vi "Func_StoreIconInfo.vi"() -> (2 "Text":T1[](array[typedef]) {"Body Text Spec"."Alignment" items=["left", "center", "right"]}, 3 "Layers":cluster{"User Layers":T5[]}[](array[cluster]) {"User Layers"."Data"."Opacity" scale=0.0..100.0})   [LabVIEW 2013]
uses:
  <vilib>/Utility/miscctls.llb/LVPoint32TypeDef.ctl
  IconEditorBuilds/2011IconEditor.llb/LayerType.ctl
  IconEditorBuilds/2011IconEditor.llb/Layer.ctl
  IconEditorBuilds/2011IconEditor.llb/User layer data.ctl
  TemplateGenerator.lvlib
  IconEditorBuilds/2011IconEditor.llb/GET Icon Text layer (VI).vi
  IconEditorBuilds/2011IconEditor.llb/GET Icon user layer (VI).vi
  IconEditorBuilds/2011IconEditor.llb/BodyText.ctl
  IconEditorBuilds/2011IconEditor.llb/Font Size.ctl
  IconEditorBuilds/2011IconEditor.llb/Alignment.ctl
  IconEditorBuilds/2011IconEditor.llb/Font.ctl
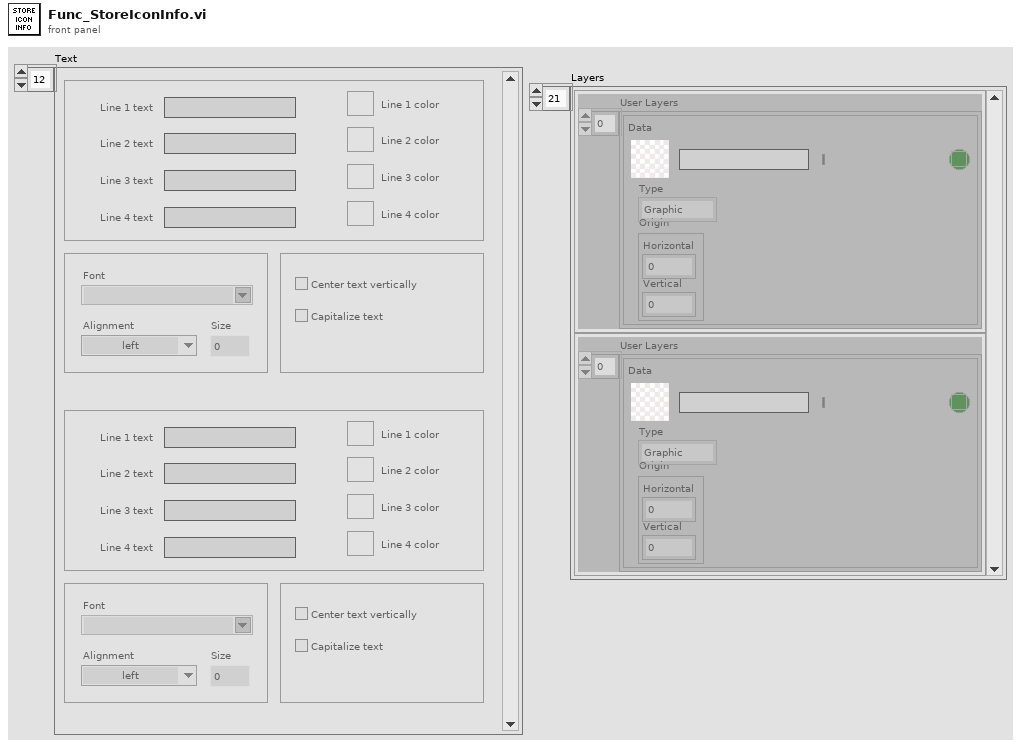
[diagram p1: front panel]
types:
  T1 = typedef "TemplateGenerator.lvlib/BodyText.ctl" = cluster{"Line 1 text":string, "Line 2 text":string, "Line 3 text":string, "Line 4 text":string, "Line 1 color":u32, "Line 2 color":u32, "Line 3 color":u32, "Line 4 color":u32, "Body Text Spec":cluster{"Font":T2, "Alignment":T3, "Size":T4}, "Center text vertically":bool, "Capitalize Text":bool}
  T2 = typedef "TemplateGenerator.lvlib/Font.ctl" = string
  T3 = typedef "TemplateGenerator.lvlib/Alignment.ctl" = u16
  T4 = typedef "TemplateGenerator.lvlib/Font Size.ctl" = u8
  T5 = typedef "TemplateGenerator.lvlib/2011 Icon Editor API.lvlib/User layer data.ctl" = cluster{"Data":T6, "Type":T7, "Origin":T8}
  T6 = typedef "TemplateGenerator.lvlib/Layer.ctl" = cluster{"LayerIcon":picture, "LayerName":string, "Opacity":u8, "Visibility?":bool}
  T7 = typedef "TemplateGenerator.lvlib/LayerType.ctl" = enum16{"Graphic", "Text", "Tool", "Graphic Drop"}
  T8 = typedef "LVPoint32TypeDef.ctl" = cluster{"Horizontal":i32, "Vertical":i32}
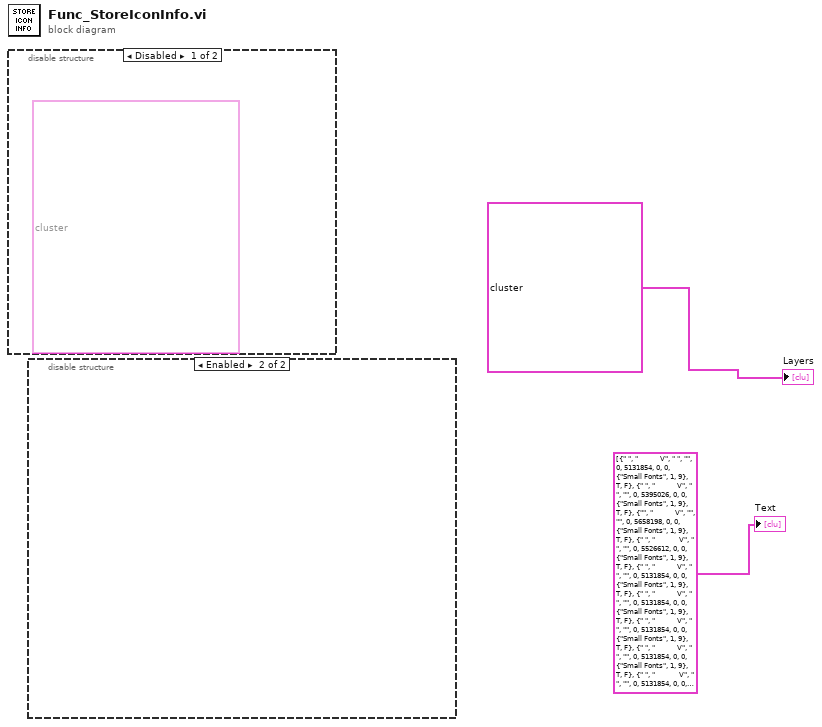
[diagram p0: block diagram]
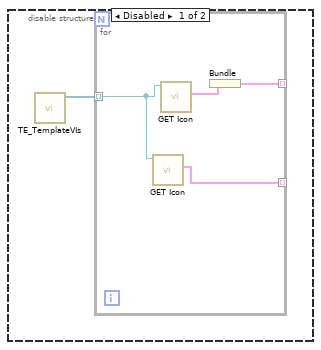
[diagram p2: hidden frame]
diagram:
  n1 = disable-structure shown="Disabled" {
    frame Disabled {
      (unwired) cluster{"User Layers":T5[], "Text 2":T1[]}[] data[207242B] ("Layers 2")
    }
    frame Enabled {
    }
  }
  n2 = disable-structure shown="Enabled" {
    frame Disabled {
      n3 = call "TE_TemplateVIs.vi"() -> ("VI References"=w3:refnum<vi>[])  [unwired: 11 in]
      n4 = for {
        tunnel: w3 -> [w7] mode=indexing
        tunnel: [w5] -> _ mode=indexing
        tunnel: [w4] -> _ mode=indexing
        n5 = call-poly "GET Icon.vi"("VI Refnum"=w7) -> ("Body Text"=w4:T1)  [unwired: 6 in, 4 out]
        n6 = call-poly "GET Icon.vi"("VI Refnum"=w7) -> ("User Layers"=w6:T5[])  [unwired: 8 in, 2 out]
        n7 = Bundle("User Layers"=w6) -> (w5:cluster{"User Layers":T5[]})  [unwired: 1 in]
      }
    }
    frame Enabled {
    }
  }
  "Layers" <- cluster{"User Layers":T5[]}[] [{"User Layers"=[{"Data"={"LayerIcon"=bytes[3230], "LayerName"="Fill", "Opacity"=100, "Visibility?"=TRUE}, "Type"=enum."Tool", "Origin"={"Horizontal"=0, "Vertical"=0}}, {"Data"={"LayerIcon"=bytes[3230], "LayerName"="path2", "Opacity"=100, "Visibility?"=TRUE}, "Type"=enum."Graphic", "Origin"={"Horizontal"=-2, "Vertical"=-2}}, {"Data"={"LayerIcon"=bytes[254], "LayerName"="Clipboard", "Opacity"=100, "Visibility?"=TRUE}, "Type"=enum."Graphic", "Origin"={"Horizontal"=-22, "Vertical"=-1}}, {"Data"={"LayerIcon"=bytes[3230], "LayerName"="flag", "Opacity"=100, "Visibility?"=TRUE}, "Type"=enum."Graphic", "Origin"={"Horizontal"=-3, "Vertical"=-10}}, {"Data"={"LayerIcon"=bytes[3230], "LayerName"="variant", "Opacity"=100, "Visibility?"=TRUE}, "Type"=enum."Graphic", "Origin"={"Horizontal"=-16, "Vertical"=-20}}, {"Data"={"LayerIcon"=bytes[2430], "LayerName"="Frame", "Opacity"=100, "Visibility?"=TRUE}, "Type"=enum."Graphic", "Origin"={"Horizontal"=0, "Vertical"=-8}}, {"Data"={"LayerIcon"=bytes[3130], "LayerName"="string node", "Opacity"=100, "Visibility?"=TRUE}, "Type"=enum."Graphic", "Origin"={"Horizontal"=0, "Vertical"=0}}]}, {"User Layers"=[{"Data"={"LayerIcon"=bytes[3230], "LayerName"="variant", "Opacity"=100, "Visibility?"=TRUE}, "Type"=enum."Graphic", "Origin"={"Horizontal"=-16, "Vertical"=-20}}, {"Data"={"LayerIcon"=bytes[3230], "LayerName"="string node", "Opacity"=100, "Visibility?"=TRUE}, "Type"=enum."Graphic", "Origin"={"Horizontal"=0, "Vertical"=0}}, {"Data"={"LayerIcon"=bytes[2430], "LayerName"="Frame", "Opacity"=100, "Visibility?"=TRUE}, "Type"=enum."Graphic", "Origin"={"Horizontal"=0, "Vertical"=-8}}]}, {"User Layers"=[{"Data"={"LayerIcon"=bytes[3230], "LayerName"="FIND2", "Opacity"=100, "Visibility?"=TRUE}, "Type"=enum."Graphic", "Origin"={"Horizontal"=-6, "Vertical"=-18}}, {"Data"={"LayerIcon"=bytes[3230], "LayerName"="variant", "Opacity"=100, "Visibility?"=TRUE}, "Type"=enum."Graphic", "Origin"={"Horizontal"=-16, "Vertical"=-20}}, {"Data"={"LayerIcon"=bytes[2430], "LayerName"="Frame", "Opacity"=100, "Visibility?"=TRUE}, "Type"=enum."Graphic", "Origin"={"Horizontal"=0, "Vertical"=-8}}, {"Data"={"LayerIcon"=bytes[3130], "LayerName"="string node", "Opacity"=100, "Visibility?"=TRUE}, "Type"=enum."Graphic", "Origin"={"Horizontal"=0, "Vertical"=0}}]}, {"User Layers"=[{"Data"={"LayerIcon"=bytes[3230], "LayerName"="Edit", "Opacity"=100, "Visibility?"=TRUE}, "Type"=enum."Graphic", "Origin"={"Horizontal"=-9, "Vertical"=-12}}, {"Data"={"LayerIcon"=bytes[3230], "LayerName"="variant", "Opacity"=100, "Visibility?"=TRUE}, "Type"=enum."Graphic", "Origin"={"Horizontal"=-16, "Vertical"=-20}}, {"Data"={"LayerIcon"=bytes[2430], "LayerName"="Frame", "Opacity"=100, "Visibility?"=TRUE}, "Type"=enum."Graphic", "Origin"={"Horizontal"=0, "Vertical"=-8}}, {"Data"={"LayerIcon"=bytes[3130], "LayerName"="string node", "Opacity"=100, "Visibility?"=TRUE}, "Type"=enum."Graphic", "Origin"={"Horizontal"=0, "Vertical"=0}}]}, {"User Layers"=[{"Data"={"LayerIcon"=bytes[3230], "LayerName"="FIND2", "Opacity"=100, "Visibility?"=TRUE}, "Type"=enum."Graphic", "Origin"={"Horizontal"=-6, "Vertical"=-18}}, {"Data"={"LayerIcon"=bytes[254], "LayerName"="Clipboard", "Opacity"=100, "Visibility?"=TRUE}, "Type"=enum."Graphic", "Origin"={"Horizontal"=0, "Vertical"=-1}}, {"Data"={"LayerIcon"=bytes[3230], "LayerName"="variant", "Opacity"=100, "Visibility?"=TRUE}, "Type"=enum."Graphic", "Origin"={"Horizontal"=-16, "Vertical"=-20}}, {"Data"={"LayerIcon"=bytes[2430], "LayerName"="Frame", "Opacity"=100, "Visibility?"=TRUE}, "Type"=enum."Graphic", "Origin"={"Horizontal"=0, "Vertical"=-8}}]}, {"User Layers"=[{"Data"={"LayerIcon"=bytes[3230], "LayerName"="Edit", "Opacity"=100, "Visibility?"=TRUE}, "Type"=enum."Graphic", "Origin"={"Horizontal"=-10, "Vertical"=-12}}, {"Data"={"LayerIcon"=bytes[254], "LayerName"="Clipboard", "Opacity"=100, "Visibility?"=TRUE}, "Type"=enum."Graphic", "Origin"={"Horizontal"=0, "Vertical"=-1}}, {"Data"={"LayerIcon"=bytes[3230], "LayerName"="variant", "Opacity"=100, "Visibility?"=TRUE}, "Type"=enum."Graphic", "Origin"={"Horizontal"=-16, "Vertical"=-20}}, {"Data"={"LayerIcon"=bytes[2430], "LayerName"="Frame", "Opacity"=100, "Visibility?"=TRUE}, "Type"=enum."Graphic", "Origin"={"Horizontal"=0, "Vertical"=-8}}]}, {"User Layers"=[{"Data"={"LayerIcon"=bytes[3230], "LayerName"="Fill", "Opacity"=100, "Visibility?"=TRUE}, "Type"=enum."Tool", "Origin"={"Horizontal"=0, "Vertical"=0}}, {"Data"={"LayerIcon"=bytes[3230], "LayerName"="public", "Opacity"=100, "Visibility?"=TRUE}, "Type"=enum."Graphic", "Origin"={"Horizontal"=-1, "Vertical"=-1}}, {"Data"={"LayerIcon"=bytes[254], "LayerName"="Clipboard", "Opacity"=100, "Visibility?"=TRUE}, "Type"=enum."Graphic", "Origin"={"Horizontal"=0, "Vertical"=-1}}, {"Data"={"LayerIcon"=bytes[3230], "LayerName"="flag", "Opacity"=100, "Visibility?"=TRUE}, "Type"=enum."Graphic", "Origin"={"Horizontal"=-14, "Vertical"=-16}}, {"Data"={"LayerIcon"=bytes[3230], "LayerName"="FIND2", "Opacity"=100, "Visibility?"=TRUE}, "Type"=enum."Graphic", "Origin"={"Horizontal"=-6, "Vertical"=-18}}, {"Data"={"LayerIcon"=bytes[3230], "LayerName"="VI Icon", "Opacity"=100, "Visibility?"=FALSE}, "Type"=enum."Graphic", "Origin"={"Horizontal"=0, "Vertical"=0}}, {"Data"={"LayerIcon"=bytes[2430], "LayerName"="Frame", "Opacity"=100, "Visibility?"=TRUE}, "Type"=enum."Graphic", "Origin"={"Horizontal"=0, "Vertical"=-8}}]}, {"User Layers"=[{"Data"={"LayerIcon"=bytes[3230], "LayerName"="Fill", "Opacity"=100, "Visibility?"=TRUE}, "Type"=enum."Tool", "Origin"={"Horizontal"=0, "Vertical"=0}}, {"Data"={"LayerIcon"=bytes[3230], "LayerName"="public", "Opacity"=100, "Visibility?"=TRUE}, "Type"=enum."Graphic", "Origin"={"Horizontal"=-1, "Vertical"=-1}}, {"Data"={"LayerIcon"=bytes[254], "LayerName"="Clipboard", "Opacity"=100, "Visibility?"=TRUE}, "Type"=enum."Graphic", "Origin"={"Horizontal"=0, "Vertical"=-1}}, {"Data"={"LayerIcon"=bytes[3230], "LayerName"="flag", "Opacity"=100, "Visibility?"=TRUE}, "Type"=enum."Graphic", "Origin"={"Horizontal"=-13, "Vertical"=-16}}, {"Data"={"LayerIcon"=bytes[3230], "LayerName"="Edit", "Opacity"=100, "Visibility?"=TRUE}, "Type"=enum."Graphic", "Origin"={"Horizontal"=-10, "Vertical"=-12}}, {"Data"={"LayerIcon"=bytes[2430], "LayerName"="Frame", "Opacity"=100, "Visibility?"=TRUE}, "Type"=enum."Graphic", "Origin"={"Horizontal"=0, "Vertical"=-8}}]}, {"User Layers"=[{"Data"={"LayerIcon"=bytes[3230], "LayerName"="variant", "Opacity"=100, "Visibility?"=TRUE}, "Type"=enum."Graphic", "Origin"={"Horizontal"=0, "Vertical"=0}}, {"Data"={"LayerIcon"=bytes[3230], "LayerName"="variant", "Opacity"=100, "Visibility?"=TRUE}, "Type"=enum."Graphic", "Origin"={"Horizontal"=0, "Vertical"=0}}, {"Data"={"LayerIcon"=bytes[3230], "LayerName"="variant", "Opacity"=100, "Visibility?"=TRUE}, "Type"=enum."Graphic", "Origin"={"Horizontal"=0, "Vertical"=0}}, {"Data"={"LayerIcon"=bytes[3230], "LayerName"="FIND2", "Opacity"=100, "Visibility?"=TRUE}, "Type"=enum."Graphic", "Origin"={"Horizontal"=-6, "Vertical"=-18}}, {"Data"={"LayerIcon"=bytes[2430], "LayerName"="Frame", "Opacity"=100, "Visibility?"=TRUE}, "Type"=enum."Graphic", "Origin"={"Horizontal"=0, "Vertical"=-8}}, {"Data"={"LayerIcon"=bytes[3130], "LayerName"="string node", "Opacity"=100, "Visibility?"=TRUE}, "Type"=enum."Graphic", "Origin"={"Horizontal"=0, "Vertical"=0}}]}, {"User Layers"=[{"Data"={"LayerIcon"=bytes[3230], "LayerName"="variant", "Opacity"=100, "Visibility?"=TRUE}, "Type"=enum."Graphic", "Origin"={"Horizontal"=0, "Vertical"=0}}, {"Data"={"LayerIcon"=bytes[3230], "LayerName"="variant", "Opacity"=100, "Visibility?"=TRUE}, "Type"=enum."Graphic", "Origin"={"Horizontal"=0, "Vertical"=0}}, {"Data"={"LayerIcon"=bytes[3230], "LayerName"="variant", "Opacity"=100, "Visibility?"=TRUE}, "Type"=enum."Graphic", "Origin"={"Horizontal"=0, "Vertical"=0}}, {"Data"={"LayerIcon"=bytes[3230], "LayerName"="Edit", "Opacity"=100, "Visibility?"=TRUE}, "Type"=enum."Graphic", "Origin"={"Horizontal"=-8, "Vertical"=-12}}, {"Data"={"LayerIcon"=bytes[2430], "LayerName"="Frame", "Opacity"=100, "Visibility?"=TRUE}, "Type"=enum."Graphic", "Origin"={"Horizontal"=0, "Vertical"=-8}}, {"Data"={"LayerIcon"=bytes[3130], "LayerName"="string node", "Opacity"=100, "Visibility?"=TRUE}, "Type"=enum."Graphic", "Origin"={"Horizontal"=0, "Vertical"=0}}]}, {"User Layers"=[{"Data"={"LayerIcon"=bytes[399], "LayerName"="namelist", "Opacity"=100, "Visibility?"=TRUE}, "Type"=enum."Graphic", "Origin"={"Horizontal"=-15, "Vertical"=-19}}, {"Data"={"LayerIcon"=bytes[2430], "LayerName"="Frame", "Opacity"=100, "Visibility?"=TRUE}, "Type"=enum."Graphic", "Origin"={"Horizontal"=0, "Vertical"=-8}}, {"Data"={"LayerIcon"=bytes[3130], "LayerName"="string node", "Opacity"=100, "Visibility?"=TRUE}, "Type"=enum."Graphic", "Origin"={"Horizontal"=0, "Vertical"=0}}]}, {"User Layers"=[{"Data"={"LayerIcon"=bytes[3232], "LayerName"="VI Icon", "Opacity"=100, "Visibility?"=TRUE}, "Type"=enum."Graphic", "Origin"={"Horizontal"=0, "Vertical"=0}}]}, {"User Layers"=[{"Data"={"LayerIcon"=bytes[3232], "LayerName"="VI Icon", "Opacity"=100, "Visibility?"=TRUE}, "Type"=enum."Graphic", "Origin"={"Horizontal"=0, "Vertical"=0}}]}, {"User Layers"=[{"Data"={"LayerIcon"=bytes[3232], "LayerName"="VI Icon", "Opacity"=100, "Visibility?"=TRUE}, "Type"=enum."Graphic", "Origin"={"Horizontal"=0, "Vertical"=0}}]}, {"User Layers"=[{"Data"={"LayerIcon"=bytes[3232], "LayerName"="VI Icon", "Opacity"=100, "Visibility?"=TRUE}, "Type"=enum."Graphic", "Origin"={"Horizontal"=0, "Vertical"=0}}]}, {"User Layers"=[{"Data"={"LayerIcon"=bytes[3232], "LayerName"="VI Icon", "Opacity"=100, "Visibility?"=TRUE}, "Type"=enum."Graphic", "Origin"={"Horizontal"=0, "Vertical"=0}}]}, {"User Layers"=[{"Data"={"LayerIcon"=bytes[3232], "LayerName"="VI Icon", "Opacity"=100, "Visibility?"=TRUE}, "Type"=enum."Graphic", "Origin"={"Horizontal"=0, "Vertical"=0}}]}, {"User Layers"=[{"Data"={"LayerIcon"=bytes[3230], "LayerName"="path2", "Opacity"=100, "Visibility?"=TRUE}, "Type"=enum."Graphic", "Origin"={"Horizontal"=-2, "Vertical"=-2}}, {"Data"={"LayerIcon"=bytes[254], "LayerName"="indexgen", "Opacity"=100, "Visibility?"=TRUE}, "Type"=enum."Graphic", "Origin"={"Horizontal"=-22, "Vertical"=-1}}, {"Data"={"LayerIcon"=bytes[3230], "LayerName"="variant", "Opacity"=100, "Visibility?"=TRUE}, "Type"=enum."Graphic", "Origin"={"Horizontal"=-16, "Vertical"=-20}}, {"Data"={"LayerIcon"=bytes[2430], "LayerName"="Frame", "Opacity"=100, "Visibility?"=TRUE}, "Type"=enum."Graphic", "Origin"={"Horizontal"=0, "Vertical"=-8}}, {"Data"={"LayerIcon"=bytes[3130], "LayerName"="string node", "Opacity"=100, "Visibility?"=TRUE}, "Type"=enum."Graphic", "Origin"={"Horizontal"=0, "Vertical"=0}}]}, {"User Layers"=[{"Data"={"LayerIcon"=bytes[3232], "LayerName"="VI Icon", "Opacity"=100, "Visibility?"=TRUE}, "Type"=enum."Graphic", "Origin"={"Horizontal"=0, "Vertical"=0}}]}, {"User Layers"=[{"Data"={"LayerIcon"=bytes[3230], "LayerName"="connect", "Opacity"=100, "Visibility?"=TRUE}, "Type"=enum."Graphic", "Origin"={"Horizontal"=-11, "Vertical"=-2}}, {"Data"={"LayerIcon"=bytes[3230], "LayerName"="FIND2", "Opacity"=100, "Visibility?"=TRUE}, "Type"=enum."Graphic", "Origin"={"Horizontal"=-6, "Vertical"=-18}}, {"Data"={"LayerIcon"=bytes[3230], "LayerName"="variant", "Opacity"=100, "Visibility?"=TRUE}, "Type"=enum."Graphic", "Origin"={"Horizontal"=-16, "Vertical"=-20}}, {"Data"={"LayerIcon"=bytes[2830], "LayerName"="Frame", "Opacity"=100, "Visibility?"=TRUE}, "Type"=enum."Graphic", "Origin"={"Horizontal"=0, "Vertical"=-8}}, {"Data"={"LayerIcon"=bytes[3130], "LayerName"="string node", "Opacity"=100, "Visibility?"=TRUE}, "Type"=enum."Graphic", "Origin"={"Horizontal"=0, "Vertical"=0}}]}, {"User Layers"=[{"Data"={"LayerIcon"=bytes[3230], "LayerName"="connect", "Opacity"=100, "Visibility?"=TRUE}, "Type"=enum."Graphic", "Origin"={"Horizontal"=-10, "Vertical"=-2}}, {"Data"={"LayerIcon"=bytes[3230], "LayerName"="Edit", "Opacity"=100, "Visibility?"=TRUE}, "Type"=enum."Graphic", "Origin"={"Horizontal"=-9, "Vertical"=-12}}, {"Data"={"LayerIcon"=bytes[3230], "LayerName"="variant", "Opacity"=100, "Visibility?"=TRUE}, "Type"=enum."Graphic", "Origin"={"Horizontal"=-16, "Vertical"=-20}}, {"Data"={"LayerIcon"=bytes[2430], "LayerName"="Frame", "Opacity"=100, "Visibility?"=TRUE}, "Type"=enum."Graphic", "Origin"={"Horizontal"=0, "Vertical"=-8}}, {"Data"={"LayerIcon"=bytes[3130], "LayerName"="string node", "Opacity"=100, "Visibility?"=TRUE}, "Type"=enum."Graphic", "Origin"={"Horizontal"=0, "Vertical"=0}}]}, {"User Layers"=[{"Data"={"LayerIcon"=bytes[3230], "LayerName"="Fill", "Opacity"=100, "Visibility?"=TRUE}, "Type"=enum."Tool", "Origin"={"Horizontal"=0, "Vertical"=0}}, {"Data"={"LayerIcon"=bytes[3230], "LayerName"="string", "Opacity"=100, "Visibility?"=TRUE}, "Type"=enum."Graphic", "Origin"={"Horizontal"=-15, "Vertical"=-1}}, {"Data"={"LayerIcon"=bytes[3230], "LayerName"="variant", "Opacity"=100, "Visibility?"=TRUE}, "Type"=enum."Graphic", "Origin"={"Horizontal"=-16, "Vertical"=-20}}, {"Data"={"LayerIcon"=bytes[2430], "LayerName"="Frame", "Opacity"=100, "Visibility?"=TRUE}, "Type"=enum."Graphic", "Origin"={"Horizontal"=0, "Vertical"=-8}}, {"Data"={"LayerIcon"=bytes[3130], "LayerName"="string node", "Opacity"=100, "Visibility?"=TRUE}, "Type"=enum."Graphic", "Origin"={"Horizontal"=0, "Vertical"=0}}]}] ("Layers 3")
  "Text" <- T1[] [{"Line 1 text"=" ", "Line 2 text"="           V", "Line 3 text"=" ", "Line 4 text"="", "Line 1 color"=0, "Line 2 color"=5131854, "Line 3 color"=0, "Line 4 color"=0, "Body Text Spec"={"Font"="Small Fonts", "Alignment"=1, "Size"=9}, "Center text vertically"=TRUE, "Capitalize Text"=FALSE}, {"Line 1 text"=" ", "Line 2 text"="           V", "Line 3 text"=" ", "Line 4 text"="", "Line 1 color"=0, "Line 2 color"=5395026, "Line 3 color"=0, "Line 4 color"=0, "Body Text Spec"={"Font"="Small Fonts", "Alignment"=1, "Size"=9}, "Center text vertically"=TRUE, "Capitalize Text"=FALSE}, {"Line 1 text"="", "Line 2 text"="           V", "Line 3 text"="", "Line 4 text"="", "Line 1 color"=0, "Line 2 color"=5658198, "Line 3 color"=0, "Line 4 color"=0, "Body Text Spec"={"Font"="Small Fonts", "Alignment"=1, "Size"=9}, "Center text vertically"=TRUE, "Capitalize Text"=FALSE}, {"Line 1 text"=" ", "Line 2 text"="            V", "Line 3 text"=" ", "Line 4 text"="", "Line 1 color"=0, "Line 2 color"=5526612, "Line 3 color"=0, "Line 4 color"=0, "Body Text Spec"={"Font"="Small Fonts", "Alignment"=1, "Size"=9}, "Center text vertically"=TRUE, "Capitalize Text"=FALSE}, {"Line 1 text"=" ", "Line 2 text"="           V", "Line 3 text"=" ", "Line 4 text"="", "Line 1 color"=0, "Line 2 color"=5131854, "Line 3 color"=0, "Line 4 color"=0, "Body Text Spec"={"Font"="Small Fonts", "Alignment"=1, "Size"=9}, "Center text vertically"=TRUE, "Capitalize Text"=FALSE}, {"Line 1 text"=" ", "Line 2 text"="           V", "Line 3 text"=" ", "Line 4 text"="", "Line 1 color"=0, "Line 2 color"=5131854, "Line 3 color"=0, "Line 4 color"=0, "Body Text Spec"={"Font"="Small Fonts", "Alignment"=1, "Size"=9}, "Center text vertically"=TRUE, "Capitalize Text"=FALSE}, {"Line 1 text"=" ", "Line 2 text"="           V", "Line 3 text"=" ", "Line 4 text"="", "Line 1 color"=0, "Line 2 color"=5131854, "Line 3 color"=0, "Line 4 color"=0, "Body Text Spec"={"Font"="Small Fonts", "Alignment"=1, "Size"=9}, "Center text vertically"=TRUE, "Capitalize Text"=FALSE}, {"Line 1 text"=" ", "Line 2 text"="           V", "Line 3 text"=" ", "Line 4 text"="", "Line 1 color"=0, "Line 2 color"=5131854, "Line 3 color"=0, "Line 4 color"=0, "Body Text Spec"={"Font"="Small Fonts", "Alignment"=1, "Size"=9}, "Center text vertically"=TRUE, "Capitalize Text"=FALSE}, {"Line 1 text"=" ", "Line 2 text"="            V", "Line 3 text"=" ", "Line 4 text"="", "Line 1 color"=0, "Line 2 color"=5131854, "Line 3 color"=0, "Line 4 color"=0, "Body Text Spec"={"Font"="Small Fonts", "Alignment"=1, "Size"=9}, "Center text vertically"=TRUE, "Capitalize Text"=FALSE}, {"Line 1 text"=" ", "Line 2 text"="           V", "Line 3 text"=" ", "Line 4 text"="", "Line 1 color"=0, "Line 2 color"=5131854, "Line 3 color"=0, "Line 4 color"=0, "Body Text Spec"={"Font"="Small Fonts", "Alignment"=1, "Size"=9}, "Center text vertically"=TRUE, "Capitalize Text"=FALSE}, {"Line 1 text"=" ", "Line 2 text"="           V", "Line 3 text"=" ", "Line 4 text"="", "Line 1 color"=0, "Line 2 color"=5131854, "Line 3 color"=0, "Line 4 color"=0, "Body Text Spec"={"Font"="Small Fonts", "Alignment"=1, "Size"=9}, "Center text vertically"=TRUE, "Capitalize Text"=FALSE}, {"Line 1 text"="", "Line 2 text"="V", "Line 3 text"="Mem", "Line 4 text"="Block", "Line 1 color"=0, "Line 2 color"=0, "Line 3 color"=0, "Line 4 color"=0, "Body Text Spec"={"Font"="Small Fonts", "Alignment"=1, "Size"=9}, "Center text vertically"=FALSE, "Capitalize Text"=TRUE}, {"Line 1 text"="", "Line 2 text"="V", "Line 3 text"="Tag", "Line 4 text"="List", "Line 1 color"=0, "Line 2 color"=0, "Line 3 color"=0, "Line 4 color"=0, "Body Text Spec"={"Font"="Small Fonts", "Alignment"=1, "Size"=9}, "Center text vertically"=FALSE, "Capitalize Text"=TRUE}, {"Line 1 text"="", "Line 2 text"="Tag", "Line 3 text"="To", "Line 4 text"="Data", "Line 1 color"=0, "Line 2 color"=16777228, "Line 3 color"=0, "Line 4 color"=0, "Body Text Spec"={"Font"="Small Fonts", "Alignment"=1, "Size"=9}, "Center text vertically"=FALSE, "Capitalize Text"=TRUE}, {"Line 1 text"="", "Line 2 text"="Data", "Line 3 text"="To", "Line 4 text"="String", "Line 1 color"=0, "Line 2 color"=16777228, "Line 3 color"=0, "Line 4 color"=0, "Body Text Spec"={"Font"="Small Fonts", "Alignment"=1, "Size"=9}, "Center text vertically"=FALSE, "Capitalize Text"=TRUE}, {"Line 1 text"="", "Line 2 text"="V", "Line 3 text"="", "Line 4 text"="", "Line 1 color"=0, "Line 2 color"=16777228, "Line 3 color"=0, "Line 4 color"=0, "Body Text Spec"={"Font"="Small Fonts", "Alignment"=1, "Size"=9}, "Center text vertically"=FALSE, "Capitalize Text"=TRUE}, {"Line 1 text"="", "Line 2 text"="", "Line 3 text"="", "Line 4 text"="", "Line 1 color"=0, "Line 2 color"=5131854, "Line 3 color"=0, "Line 4 color"=0, "Body Text Spec"={"Font"="Small Fonts", "Alignment"=1, "Size"=9}, "Center text vertically"=TRUE, "Capitalize Text"=FALSE}, {"Line 1 text"=" ", "Line 2 text"="           V", "Line 3 text"=" ", "Line 4 text"="", "Line 1 color"=0, "Line 2 color"=5131854, "Line 3 color"=0, "Line 4 color"=0, "Body Text Spec"={"Font"="Small Fonts", "Alignment"=1, "Size"=9}, "Center text vertically"=TRUE, "Capitalize Text"=FALSE}, {"Line 1 text"="", "Line 2 text"="V", "Line 3 text"=" ", "Line 4 text"="", "Line 1 color"=0, "Line 2 color"=16777228, "Line 3 color"=0, "Line 4 color"=0, "Body Text Spec"={"Font"="Small Fonts", "Alignment"=1, "Size"=10}, "Center text vertically"=FALSE, "Capitalize Text"=TRUE}, {"Line 1 text"="", "Line 2 text"="           V", "Line 3 text"="", "Line 4 text"="", "Line 1 color"=0, "Line 2 color"=0, "Line 3 color"=0, "Line 4 color"=0, "Body Text Spec"={"Font"="Small Fonts", "Alignment"=1, "Size"=9}, "Center text vertically"=TRUE, "Capitalize Text"=FALSE}, {"Line 1 text"=" ", "Line 2 text"="            V", "Line 3 text"=" ", "Line 4 text"="", "Line 1 color"=0, "Line 2 color"=5526612, "Line 3 color"=0, "Line 4 color"=0, "Body Text Spec"={"Font"="Small Fonts", "Alignment"=1, "Size"=9}, "Center text vertically"=TRUE, "Capitalize Text"=FALSE}, {"Line 1 text"=" ", "Line 2 text"="           V", "Line 3 text"=" ", "Line 4 text"="", "Line 1 color"=0, "Line 2 color"=5131854, "Line 3 color"=0, "Line 4 color"=0, "Body Text Spec"={"Font"="Small Fonts", "Alignment"=1, "Size"=9}, "Center text vertically"=TRUE, "Capitalize Text"=FALSE}] ("Text 4")
